vi "SimAdc Fetch Samples.vi"(8 "error in":errorcluster, 10 "max samples per fetch (1M)":i64=1000000, 11 "simadc in":T1) -> (0 "error out":errorcluster, 1 "done":bool, 2 "sample data":i32[][](array[numeric]), 3 "simadc out":T1, 4 "samples fetched":i64, 5 "scale factor [V]":dbl, 6 "smpl offset":i64, 7 "Ts [s]":dbl)   [LabVIEW 2018]
doc: "Fetches simulated samples from the ADC."
uses:
  SimAdc Config.ctl
  SimAdc Channel Cfg.ctl
  <vilib>/Analysis/baseanly.llb/Real A x B.vi
  <vilib>/Analysis/Matrix/Numeric/Conversions/Array To Matrix - RA.vi
  <vilib>/Analysis/Matrix/Numeric/Add/Add - RM,RM.vi
  <vilib>/Analysis/Matrix/Numeric/Conversions/Matrix To Array - RM.vi
  <vilib>/Analysis/Matrix/NI_Matrix.lvlib
  <vilib>/Analysis/NI_AALBase.lvlib
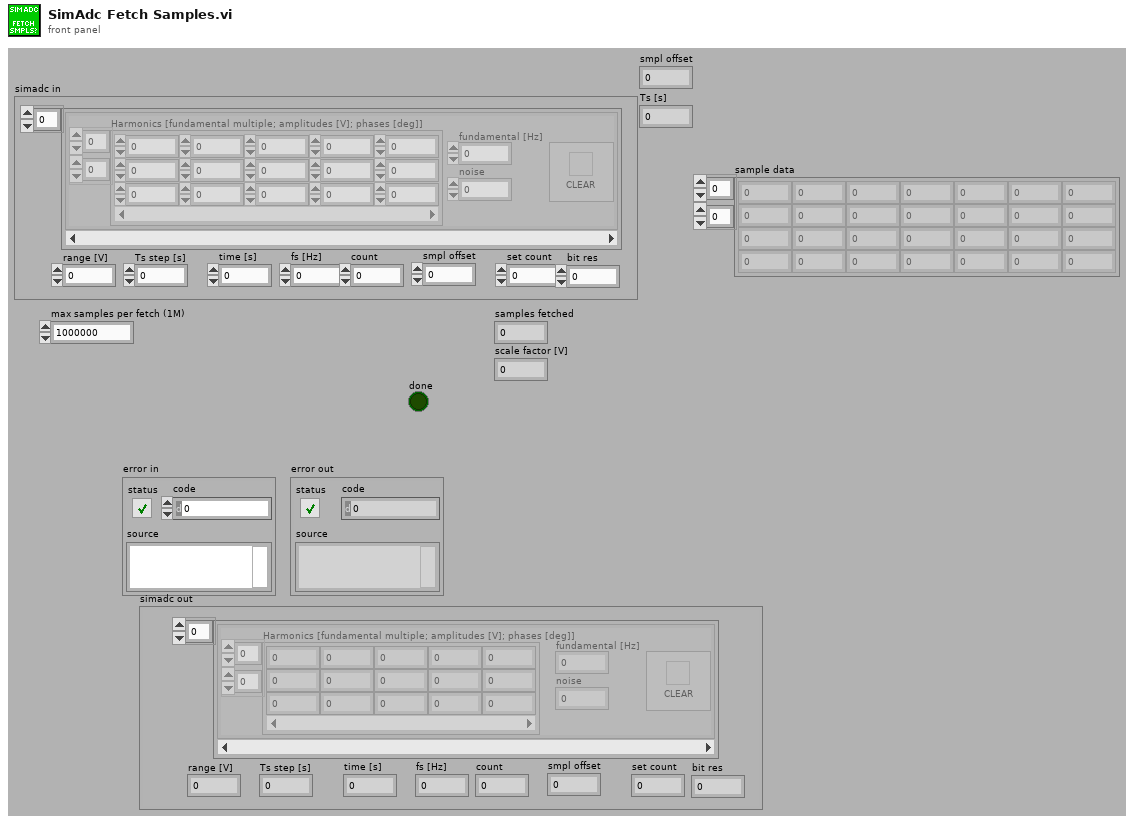
[diagram p1: front panel]
types:
  T1 = typedef "SimAdc Config.ctl" = cluster{"channels":T2[], "range [V]":dbl, "Ts step [s]":dbl, "time [s]":dbl, "fs [Hz]":dbl, "count":i64, "smpl offset":i64, "set count":i64, "bit res":i32}
  T2 = typedef "SimAdc Channel Cfg.ctl" = cluster{"harmonics":dbl[][], "btn clear":bool, "noise":dbl, "fundamental [Hz]":dbl}
  T3 = typedef "NI_Matrix.lvlib/RealMatrix.ctl" = dbl[][]
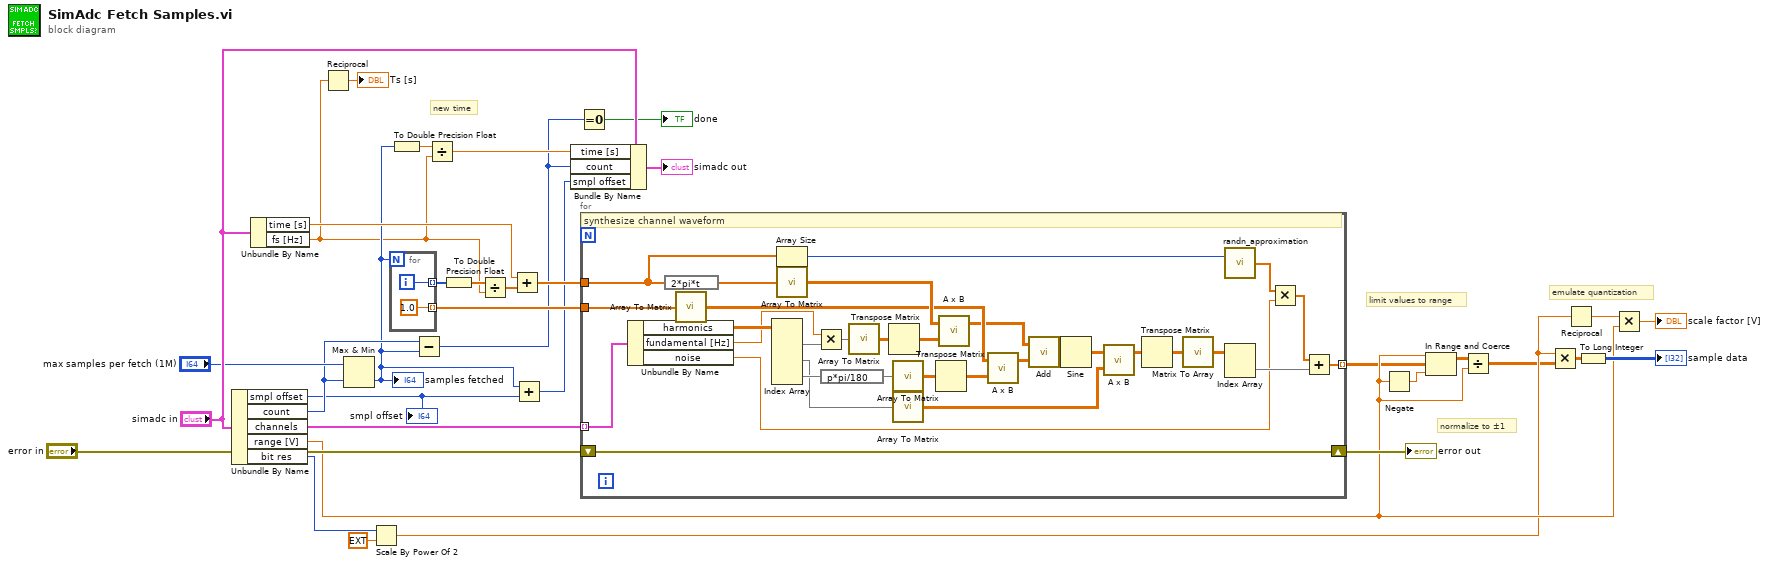
[diagram p0: block diagram]
diagram:
  # "emulate quantization"
  # "normalize to ±1"
  # "limit values to range"
  # "new time"
  n1 = Unbundle By Name("simadc in") -> ("smpl offset"=w16:i64, "count"=w21:i64, "channels"=w34:T2[], "range [V]"=w8:dbl, "bit res"=w6:i32)
  "smpl offset" <- w16
  n2 = Unbundle By Name("simadc in") -> ("time [s]"=w27:dbl, "fs [Hz]"=w13:dbl)
  n3 = Reciprocal(x=w13) -> (1/x=→"Ts [s]":dbl)
  n4 = Max & Min(x="max samples per fetch (1M)", y=w21) -> (min(x,y)=w15:i64)  [unwired: 1 out]
  "samples fetched" <- w15
  n5 = Scale By Power Of 2(n=w6, x=ext 1.0) -> (x*2^n=w4:ext)
  n6 = for {
    N: w15 -> [_]
    tunnel: [w36] -> w30 mode=indexing
    tunnel: [1.0] -> w23 mode=indexing
    i -> [w36]
  }
  n7 = To Double Precision Float(number=w15) -> (double precision float=w26:dbl)
  n8 = Subtract(x=w21, y=w15) -> (x-y=w20:i64)
  n9 = Divide(x=w26, y=w13) -> (x/y=w22:dbl)
  n10 = To Double Precision Float(number=w30) -> (double precision float=w29:dbl[])
  n11 = Divide(x=w29, y=w13) -> (x/y=w28:dbl[])
  n12 = Add(x=w27, y=w28) -> (x+y=w25:dbl[])
  n13 = Add(x=w15, y=w16) -> (x+y=w14:i64)
  n14 = Bundle By Name(cluster="simadc in", "time [s]"=w22, "count"=w20, "smpl offset"=w14) -> (→"simadc out":T1)
  n15 = Equal To 0?(x=w20) -> (x = 0?=→"done":bool)
  n16 = for {
    shift-right: [w68] -> w32
    shift-left: "error in" -> [w68]
    tunnel: w34 -> [w67] mode=indexing
    tunnel: w25 -> [w43]
    tunnel: w23 -> [w56]
    tunnel: [w40] -> w2 mode=indexing
    # "synthesize channel waveform"
    n17 = Unbundle By Name(w67) -> ("harmonics"=w66:dbl[][], "fundamental [Hz]"=w64:dbl, "noise"=w38:dbl)
    n18 = expression code="2*pi*t"(w43) -> (w61:dbl[])
    n19 = call-poly <vilib>:"Array To Matrix.vi"("Real 1D Array"=w56) -> ("Real Matrix (Column Vector)"=w54:T3)
    n20 = Index Array(array=w66) -> (element #1=w65:dbl[], element #2=w49:dbl[], element #3=w58:dbl[])  [unwired: 6 in]
    n21 = Array Size(array=w43) -> (size(s)=w42:i32)
    n22 = call-poly <vilib>:"Array To Matrix.vi"("Real 1D Array"=w61) -> ("Real Matrix (Column Vector)"=w59:T3)
    n23 = Multiply(x=w64, y=w65) -> (x*y=w63:dbl[])
    n24 = expression code="p*pi/180"(w58) -> (w57:dbl[])
    n25 = call-poly <vilib>:"Array To Matrix.vi"("Real 1D Array"=w63) -> ("Real Matrix (Column Vector)"=w62:T3)
    n26 = Transpose Matrix(1:w62) -> (0:w60:T3)
    n27 = call-poly <vilib>:"Array To Matrix.vi"("Real 1D Array"=w57) -> ("Real Matrix (Column Vector)"=w55:T3)
    n28 = call-poly <vilib>:"Array To Matrix.vi"("Real 1D Array"=w49) -> ("Real Matrix (Column Vector)"=w47:T3)
    n29 = Transpose Matrix(1:w55) -> (0:w53:T3)
    n30 = call-poly <vilib>:"A x B.vi"("B"=w60, "A"=w59) -> ("A x B"=w51:T3)  [unwired: 1 out]
    n31 = call-poly <vilib>:"A x B.vi"("B"=w53, "A"=w54) -> ("A x B"=w52:T3)  [unwired: 1 out]
    n32 = call-poly <vilib>:"Add.vi"("Real Matrix B"=w52, "Real Matrix A"=w51) -> ("A + B"=w50:T3)
    n33 = Sine(x=w50) -> (sin(x)=w48:T3)
    n34 = call-poly <vilib>:"A x B.vi"("B"=w47, "A"=w48) -> ("A x B"=w46:T3)  [unwired: 1 out]
    n35 = Transpose Matrix(1:w46) -> (0:w44:T3)
    n36 = call-poly <vilib>:"Matrix To Array.vi"("Real Matrix"=w44) -> ("Real 2D Array"=w45:dbl[][])
    n37 = call "randn_approximation.vi"("N"=w42) -> ("randn() vector"=w39:dbl[])  [unwired: 1 in]
    n38 = Index Array(array=w45) -> (element=w41:dbl[])  [unwired: 2 in]
    n39 = Multiply(x=w39, y=w38) -> (x*y=w37:dbl[])
    n40 = Add(x=w37, y=w41) -> (x+y=w40:dbl[])
  }
  "error out" <- w32
  n41 = Negate(x=w8) -> (-x=w10:dbl)
  n42 = In Range and Coerce(upper limit=w8, x=w2, lower limit=w10) -> (coerced(x)=w1:dbl[][])  [unwired: 1 out]
  n43 = Divide(x=w1, y=w8) -> (x/y=w3:dbl[][])
  n44 = Multiply(x=w4, y=w3) -> (x*y=w18:ext[][])
  n45 = Reciprocal(x=w4) -> (1/x=w9:ext)
  n46 = To Long Integer(number=w18) -> (32bit integer=→"sample data":i32[][])
  n47 = Multiply(x=w9, y=w8) -> (x*y=→"scale factor [V]":ext)
